vi "Load Subject Parameters.vi"(4 "Default Parameters File":path, 5 "Subject":u16, 6 "Label.Text":string, 7 "Subject Parameters Folder":path) -> (1 "error out":errorcluster, 2 "Subject Parameters":T1 {"Subject" items=["Subject 0", "Subject 1", "Subject 2", "Subject 3", "Subject 4", "Subject 5", "Subject 6", "Subject 7", "Subject 8", "Subject 9", "Subject 10", "Subject 11", "Subject 12", "Subject 13", "Subject 14", "Subject 15", "Subject 16", "Subject 17", "Subject 18", "Subject 19", "Subject 20", "Subject 21", "Subject 22", "Subject 23", "Subject 24", "Subject 25", "Subject 26", "Subject 27", "Subject 28", "Subject 29", "Subject 30", "Subject 31", "Subject 32", "Subject 33", "Subject 34", "Subject 35", "Subject 36", "Subject 37", "Subject 38", "Subject 39", "Subject 40"]}, 3 "Source Parameter File":path)   [LabVIEW 2019]
uses:
  Controls/Subject Params.ctl
  Controls/Subject.ctl
  Controls/GPD Side Parameters.ctl
  Controls/Type Defs/Stim Parameters.ctl
  Controls/Stim off-half-ful.ctl
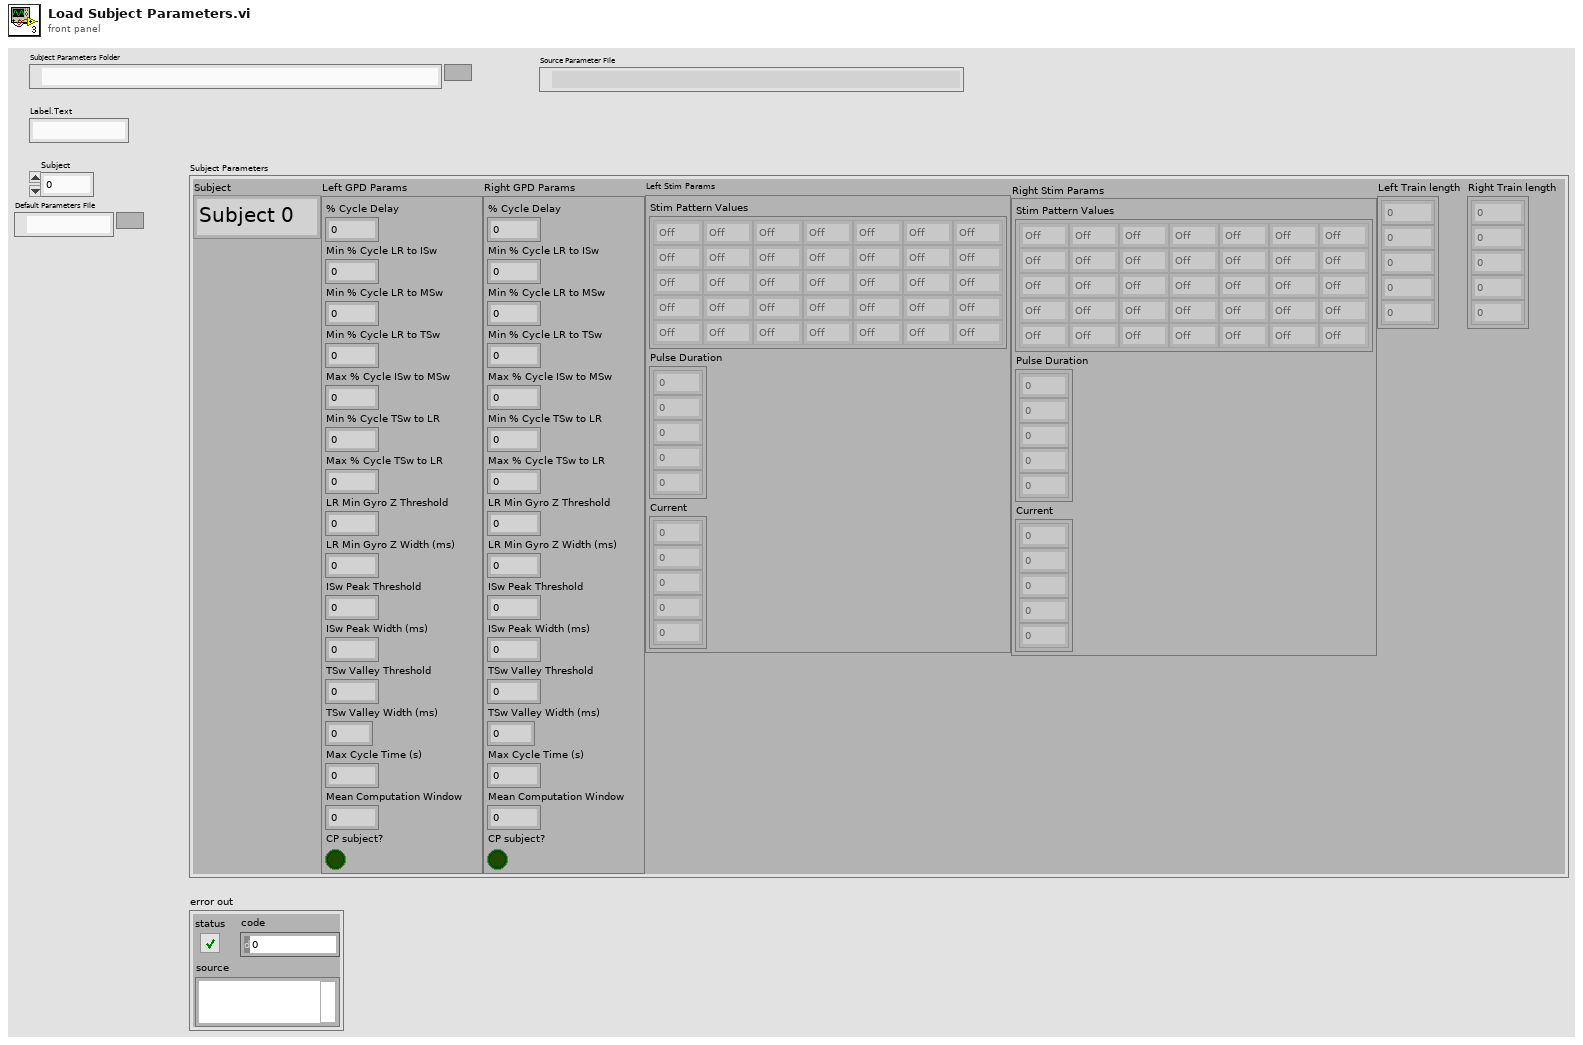
[diagram p1: front panel]
types:
  T1 = typedef "Subject Params.ctl" = cluster{"Subject":T2, "Left GPD Params":T3, "Right GPD Params":T3, "Left Stim Params":T4, "Right Stim Params":T4, "Left Train length":i64[], "Right Train length":i64[]}
  T2 = typedef "Subject.ctl" = u16
  T3 = typedef "GPD Side Parameters.ctl" = cluster{"% Cycle Delay":dbl, "Min % Cycle LR to ISw ":dbl, "Min % Cycle LR to MSw":dbl, "Min % Cycle LR to TSw":dbl, "Max % Cycle ISw to MSw":dbl, "Min % Cycle TSw to LR":dbl, "Max % Cycle TSw to LR":dbl, "LR Min Gyro Z Threshold":dbl, "LR Min Gyro Z Width":dbl, "ISw Peak Threshold":dbl, "ISw Peak Width":dbl, "TSw Valley Threshold":dbl, "TSw Valley Width (ms)":dbl, "Max Cycle Time (s)":dbl, "Mean Computation Window":dbl, "CP subject?":bool}
  T4 = typedef "Stim Parameters.ctl" = cluster{"Stim Pattern Values":T5[][], "Pulse Duration":i64[], "Current":i64[]}
  T5 = typedef "Stim off-half-ful.ctl" = enum16{"Off", "Half", "Full"}
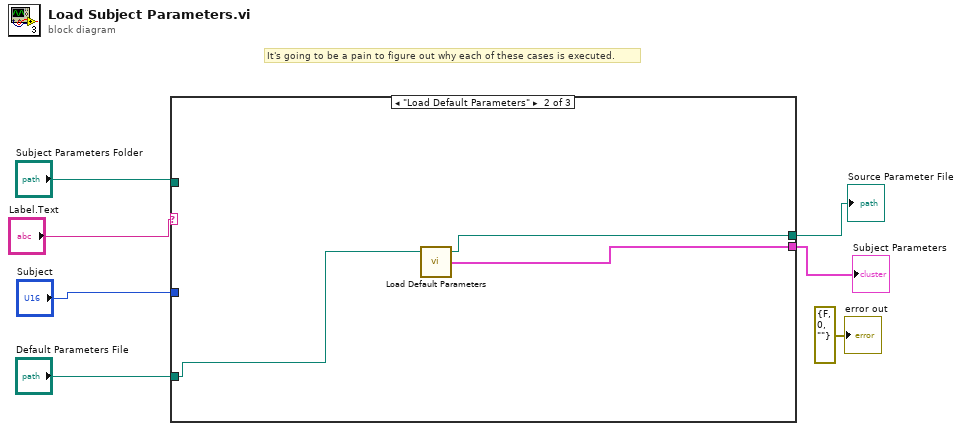
[diagram p0: block diagram]
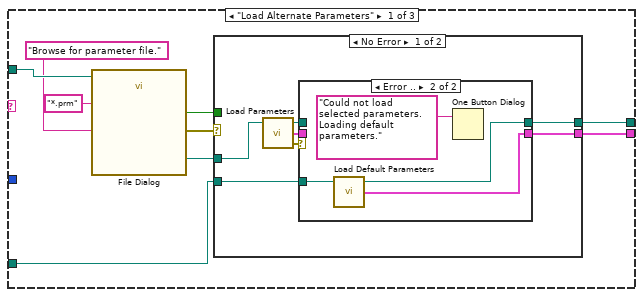
[diagram p2: hidden frame]
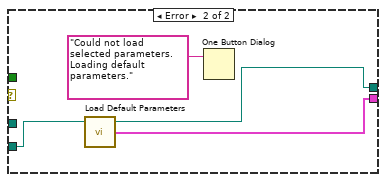
[diagram p4: hidden frame]
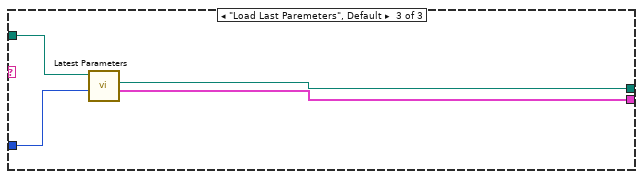
[diagram p5: hidden frame]
diagram:
  # "It's going to be a pain to figure out why each of these cases is executed."
  n1 = case shown="\"Load Default Parameters\"" "Label.Text" {
    tunnel: "Subject" -> [_ _ w40]
    tunnel: "Subject Parameters Folder" -> [w16 _ w39]
    tunnel: [w11 w34 w38] -> w4
    tunnel: [w10 w35 w37] -> w3
    tunnel: "Default Parameters File" -> [w8 w36 _]
    frame "Load Alternate Parameters" {
      n2 = call "File Dialog"("start path"=w16, "prompt"="Browse for parameter file.", "pattern (all files)"="*.prm") -> ("selected path"=w12:path, "cancelled"=w9:bool, "error out"=w13:errorcluster)  [unwired: 9 in, 1 out]
      n3 = case shown="No Error" w13 {
        tunnel: w12 -> [w23 _]
        tunnel: [w22 w30] -> w11
        tunnel: [w21 w31] -> w10
        tunnel: w9 -> [_ _]
        tunnel: w8 -> [w20 w32]
        frame No Error {
          n4 = call "Load Parameters.vi"("Subject Parameters File"=w23) -> ("error out"=w19:errorcluster, "Subject Parameters"=w17:T1, "Subject Parameters File"=w18:path)  [unwired: 2 in]
          n5 = case shown="Error .." w19 {
            tunnel: w18 -> [w24 _]
            tunnel: w17 -> [w25 _]
            tunnel: [w25 w26] -> w22
            tunnel: [w24 w27] -> w21
            tunnel: w20 -> [_ w28]
            frame No Error {
            }
            frame Error {
              n6 = call "Load Default Parameters.vi"("Default parameters file"=w28) -> ("Subject Parameters"=w26:T1, "Subject Parameters File"=w27:path)  [unwired: 3 in]
              n7 = One Button Dialog(message="Could not load selected parameters. Loading default parameters.") -> ()  [unwired: 1 in, 1 out]
            }
          }
        }
        frame Error {
          n8 = call "Load Default Parameters.vi"("Default parameters file"=w32) -> ("Subject Parameters"=w30:T1, "Subject Parameters File"=w31:path)  [unwired: 3 in]
          n9 = One Button Dialog(message="Could not load selected parameters. Loading default parameters.") -> ()  [unwired: 1 in, 1 out]
        }
      }
    }
    frame "Load Default Parameters" {
      n10 = call "Load Default Parameters.vi"("Default parameters file"=w36) -> ("Subject Parameters"=w34:T1, "Subject Parameters File"=w35:path)  [unwired: 3 in]
    }
    frame "Load Last Paremeters", Default {
      n11 = call "Latest Parameters.vi"("Subject Number"=w40, "Subject Parameters Folder"=w39) -> ("Subject Parameters"=w38:T1, "Source Parameter File"=w37:path)  [unwired: 2 in, 2 out]
    }
  }
  "Subject Parameters" <- w4
  "Source Parameter File" <- w3
  "error out" <- errorcluster {"status"=FALSE, "code"=0, "source"=""} ("error out")
